vi "IOV refnum from old URL.vi"(8 "error in (no error)":errorcluster, 11 "variable path (URL)":string) -> (0 "error out":errorcluster, 3 "IOV refnum":refnum<k21>)   [LabVIEW 2020]
uses:
  <vilib>/variable/dynamicAPI/NI_VariableDynamic.lvlib
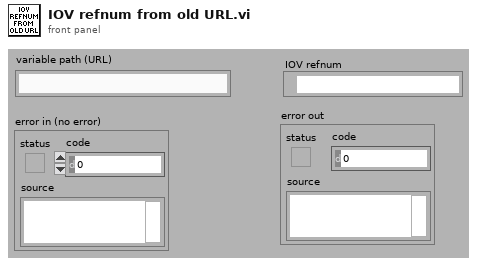
[diagram p1: front panel]
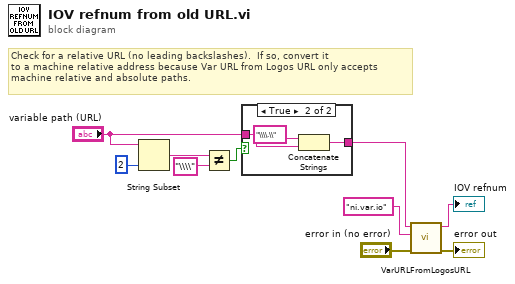
[diagram p0: block diagram]
diagram:
  # "Check for a relative URL (no leading backslashes).  If so, convert it\nto a machine relative address because Var URL from Logos URL only accepts\nmachine relative and absolute paths."
  n1 = String Subset(string="variable path (URL)", length (rest)=2 ("length (rest)")) -> (substring=w5:string)  [unwired: 1 in]
  n2 = Not Equal?(x=w5, y="\\\\") -> (x != y?=w3:bool)
  n3 = case shown="True" w3 {
    tunnel: "variable path (URL)" -> [w11 w12]
    tunnel: [w11 w14] -> w1
    frame False {
    }
    frame True {
      n4 = Concatenate Strings("\\\\.\\" ("string"), w12) -> (w14:string)
    }
  }
  n5 = call <vilib>:"VarURLFromLogosURL.vi"("error in (no error)"="error in (no error)", "scheme"="ni.var.io", "logosURL"=w1) -> ("error out"=→"error out":errorcluster, "variable URL"=→"IOV refnum":string)  [unwired: 7 in]
